vi "Eco LN2.vi"(8 "error in (no error)":errorcluster caption="Fehler (Eingang, kein Fehler)", 9 "DO 0-31":T1, 11 "Zustand cRIO":T2) -> (0 "error out":errorcluster caption="Fehler (Ausgang)", 1 "DO 0-31":T1)   [LabVIEW 2020, in "Allgemein.lvlib"]
uses:
  Allgemein.lvlib
  Verwaltung/Digital Ausgaenge 0-31.ctl
  Funktionstasten/Zustaende.ctl
  Aktion FGV Komm Systemeinstellungen.ctl
  Funktionstasten/Funktionstasten.lvlib
  Aktionen FGV Dichtheitstest.ctl
  Verwaltung/Verwaltung - cRIO.lvlib
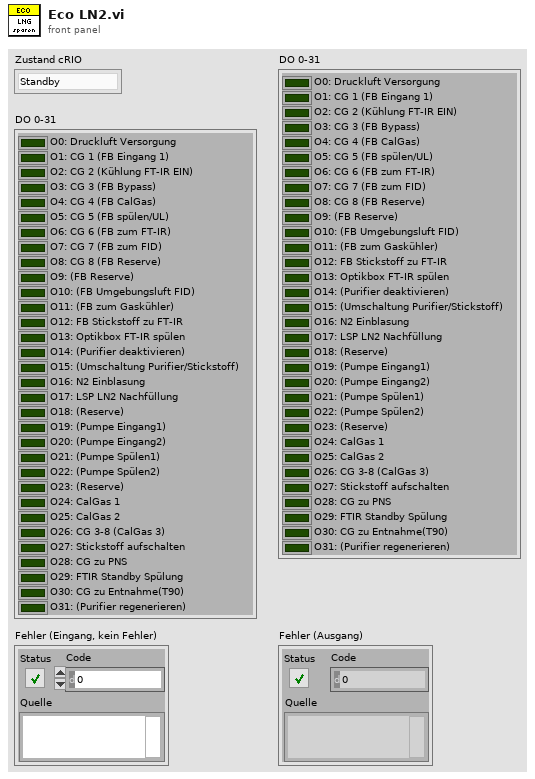
[diagram p1: front panel]
types:
  T1 = typedef "Verwaltung - cRIO.lvlib/Digital Ausgaenge 0-31.ctl" = cluster{"O0: Druckluft Versorgung":bool, "O1: CG 1 (FB Eingang 1)":bool, "O2: CG 2 (Kühlung FT-IR EIN)":bool, "O3: CG 3 (FB Bypass)":bool, "O4: CG 4 (FB CalGas)":bool, "O5: CG 5 (FB spülen/UL)":bool, "O6: CG 6 (FB zum FT-IR)":bool, "O7: CG 7 (FB zum FID)":bool, "O8: CG 8 (FB Reserve)":bool, "O9: (FB Reserve)":bool, "O10: (FB Umgebungsluft FID)":bool, "O11: (FB zum Gaskühler)":bool, "O12: FB Stickstoff zu FT-IR":bool, "O13: Optikbox FT-IR spülen":bool, "O14: (Purifier deaktivieren)":bool, "O15: (Umschaltung Purifier/Stickstoff)":bool, "O16: N2 Einblasung":bool, "O17: LSP LN2 Nachfüllung":bool, "O18: (Reserve)":bool, "O19: (Pumpe Eingang1)":bool, "O20: (Pumpe Eingang2)":bool, "O21: (Pumpe Spülen1)":bool, "O22: (Pumpe Spülen2)":bool, "O23: (Reserve)":bool, "O24: CalGas 1":bool, "O25: CalGas 2":bool, "O26: CG 3-8 (CalGas 3)":bool, "O27: Stickstoff aufschalten":bool, "O28: CG zu PNS":bool, "O29: FTIR Standby Spülung":bool, "O30: CG zu Entnahme(T90)":bool, "O31: (Purifier regenerieren)":bool}
  T2 = typedef "Funktionstasten.lvlib/Zustaende.ctl" = enum16{"Standby", "Pause", "Eco", "Messen", "Kalibrieren", "Spülen Filter", "Spülen Leitung", "Umgebungsluft", "0-Gas", "Cal-Gas", "CG zu PNS", "-------------", "Init 1", "Init 2", "Init 3", "Init 4", "Messen vorbereiten", "Messen durchführen", "Exit"}
  T3 = typedef "Allgemein.lvlib/Aktionen FGV Dichtheitstest.ctl" = enum16{"lesen", "schreiben"}
  T4 = typedef "Allgemein.lvlib/Aktion FGV Komm Systemeinstellungen.ctl" = enum16{"lesen", "schreiben"}
  T5 = typedef "Allgemein.lvlib/Cluster Komm Systemeinstellungen.ctl" = cluster{"ECO LNG":bool}
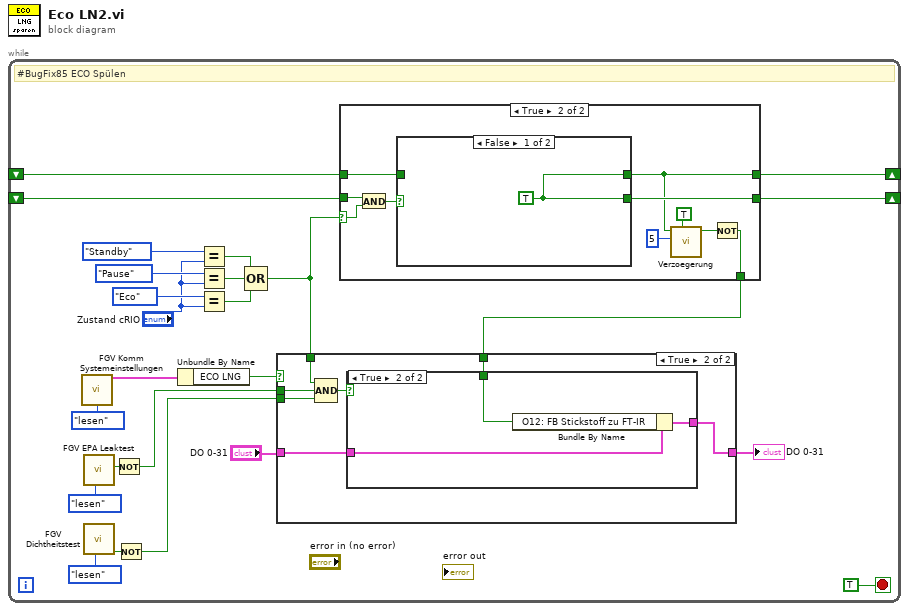
[diagram p0: block diagram]
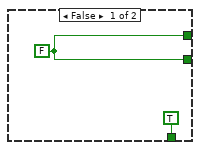
[diagram p2: hidden frame]
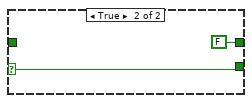
[diagram p3: hidden frame]
diagram:
  n1 = while {
    shift-right: [w11] -> _
    shift-left: _ -> [w10]
    shift-right: [w9] -> _
    shift-left: _ -> [w8]
    stop <- TRUE stop-if-true
    # "#BugFix85 ECO Spülen"
    n2 = call "FGV Komm Systemeinstellungen.vi"("Aktion"=Aktion_FGV_Komm_Systemeinstellungen."lesen") -> ("Systemeinstellungen"=w17:T5)  [unwired: 13 in, 1 out]
    n3 = call "FGV EPA Leaktest.vi"("Aktion"=enum16{"lesen", "schreiben"}."lesen") -> ("Leaktest aktiv"=w2:bool)  [unwired: 9 in, 1 out]
    n4 = call "FGV Dichtheitstest.vi"("Aktionen"=Aktionen_FGV_Dichtheitstest."lesen") -> ("Dichtheitstest?"=w5:bool)  [unwired: 9 in, 1 out]
    n5 = Not(x=w2) -> (.not. x?=w1:bool)
    n6 = Not(x=w5) -> (.not. x?=w4:bool)
    n7 = Unbundle By Name(w17) -> ("ECO LNG"=w15:bool)
    n8 = Equal?(x=Zustaende."Standby" ("Zustand cRIO"), y="Zustand cRIO") -> (x = y?=w21:bool)
    n9 = Equal?(x=Zustaende."Pause" ("Zustand cRIO"), y="Zustand cRIO") -> (x = y?=w20:bool)
    n10 = Equal?(x=Zustaende."Eco" ("Zustand cRIO"), y="Zustand cRIO") -> (x = y?=w19:bool)
    n11 = Compound Arithmetic op=OR ("Mehrfacharithmetik")(w21, w20, w19) -> (w12:bool)
    n12 = case shown="True" w12 {
      selector: w12 -> [_ w36]
      tunnel: [w27 w34] -> w9
      tunnel: [w27 w32] -> w11
      tunnel: w8 -> [_ w37]
      tunnel: w10 -> [_ w31]
      tunnel: [TRUE ("Zeit abgelaufen?") w29] -> w7
      frame False {
        w27 = FALSE
      }
      frame True {
        n13 = And(x=w37, y=w36) -> (x .and. y?=w35:bool)
        n14 = case shown="False" w35 {
          selector: w35 -> [_ w40]
          tunnel: [w38 w40] -> w34
          tunnel: [w38 FALSE ("Abfallverzögerung?")] -> w32
          tunnel: w31 -> [_ _]
          frame False {
            w38 = TRUE ("Abfallverzögerung?")
          }
          frame True {
          }
        }
        n15 = call "Verzoegerung.vi"("Abfallverzögerung?"=TRUE, "min"=u16 5, "Startsignal"=w32) -> ("Zeit abgelaufen?"=w30:bool)  [unwired: 7 in, 1 out]
        n16 = Not(x=w30) -> (.not. x?=w29:bool)
      }
    }
    n17 = case shown="True" w15 {
      tunnel: "DO 0-31" -> [w41 w48]
      tunnel: [w41 w47] -> w13
      tunnel: w7 -> [_ w46]
      tunnel: w12 -> [_ w45]
      tunnel: w4 -> [_ w43]
      tunnel: w1 -> [_ w42]
      frame False {
      }
      frame True {
        n18 = Compound Arithmetic op=AND ("Mehrfacharithmetik")(w45, w42, w43) -> (w44:bool)
        n19 = case shown="True" w44 {
          tunnel: w48 -> [w49 w52]
          tunnel: [w49 w51] -> w47
          tunnel: w46 -> [_ w50]
          frame False {
          }
          frame True {
            n20 = Bundle By Name(cluster=w52, "O12: FB Stickstoff zu FT-IR"=w50) -> (w51:T1)
          }
        }
      }
    }
    "DO 0-31" <- w13
  }
